vi "Get AccessType.vi"(8 "Error In":errorcluster, 11 "reference in":refnum<class "OD Entry.lvclass">) -> (0 "Error Out":errorcluster, 2 "AccessType":T1(ring)=enum."const", 3 "reference out":refnum<class "OD Entry.lvclass">)   [LabVIEW 2019, in "Electronic Datasheet.lvlib" / "OD Entry.lvclass"]
uses:
  OD Entry.lvclass
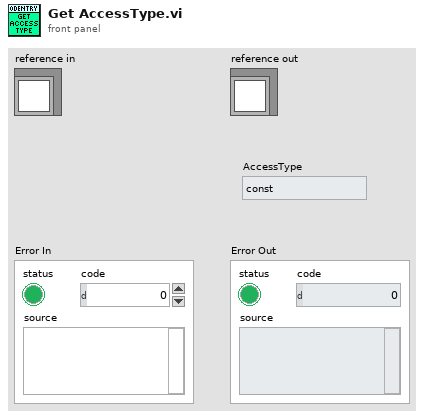
[diagram p1: front panel]
types:
  T1 = enum16{"ro", "wo", "rw", "rwr", "rww", "const", "UNKNOWN"}
  T2 = typedef "Electronic Datasheet.lvlib/Access Type.ctl" = enum16{"ro", "wo", "rw", "rwr", "rww", "const"}
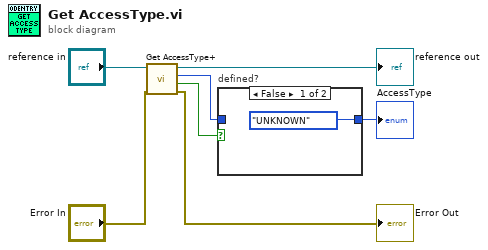
[diagram p0: block diagram]
diagram:
  n1 = call "Get AccessType+.vi"("Error In"="Error In", "reference in"="reference in") -> ("Error Out"=→"Error Out":errorcluster, "Defined?"=w3:bool, "AccessType"=w2:T2, "reference out"=→"reference out":refnum<class "OD Entry.lvclass">)  [unwired: 6 in]
  n2 = case "defined?" shown="False" w3 {
    tunnel: w2 -> [_ w9]
    tunnel: [T1."UNKNOWN" ("AccessType") w9] -> w1
    frame False {
    }
    frame True {
    }
  }
  "AccessType" <- w1
